vi "shift odd lines by.vi"(5 "calculate squared difference":bool, 7 "shift odd lines by":i32, 11 "frame in":dbl[][](array[numeric])) -> (2 "squared difference":dbl, 3 "shifted frame out":dbl[][](array[numeric]))   [LabVIEW 2012]
panel:
  out "corrected":T1(plugin-control)
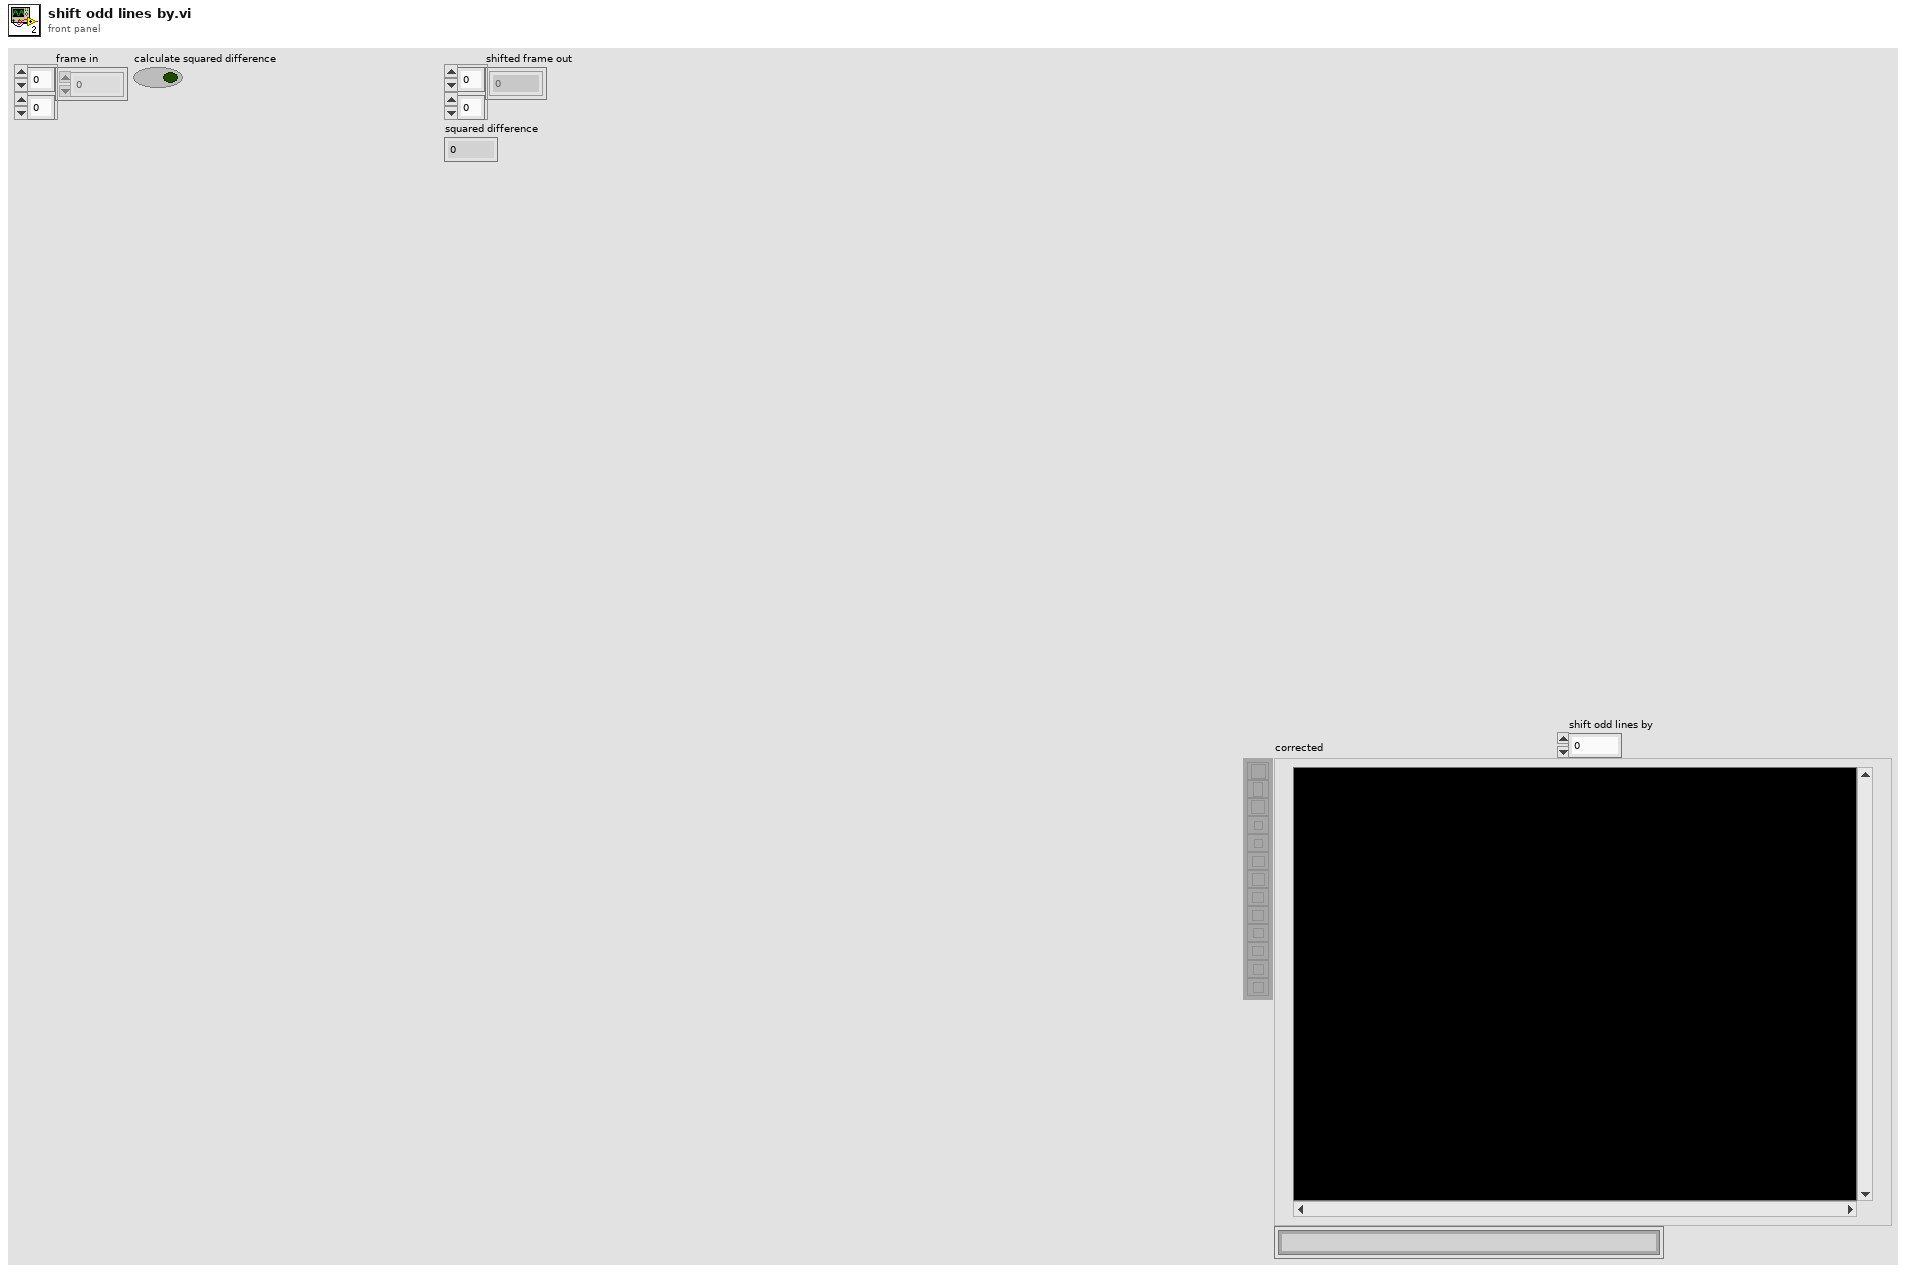
[diagram p1: front panel]
types:
  T1 = typedef "IMAQ Image.ctl" = refnum<image>
  T2 = typedef "Image Type" = u32
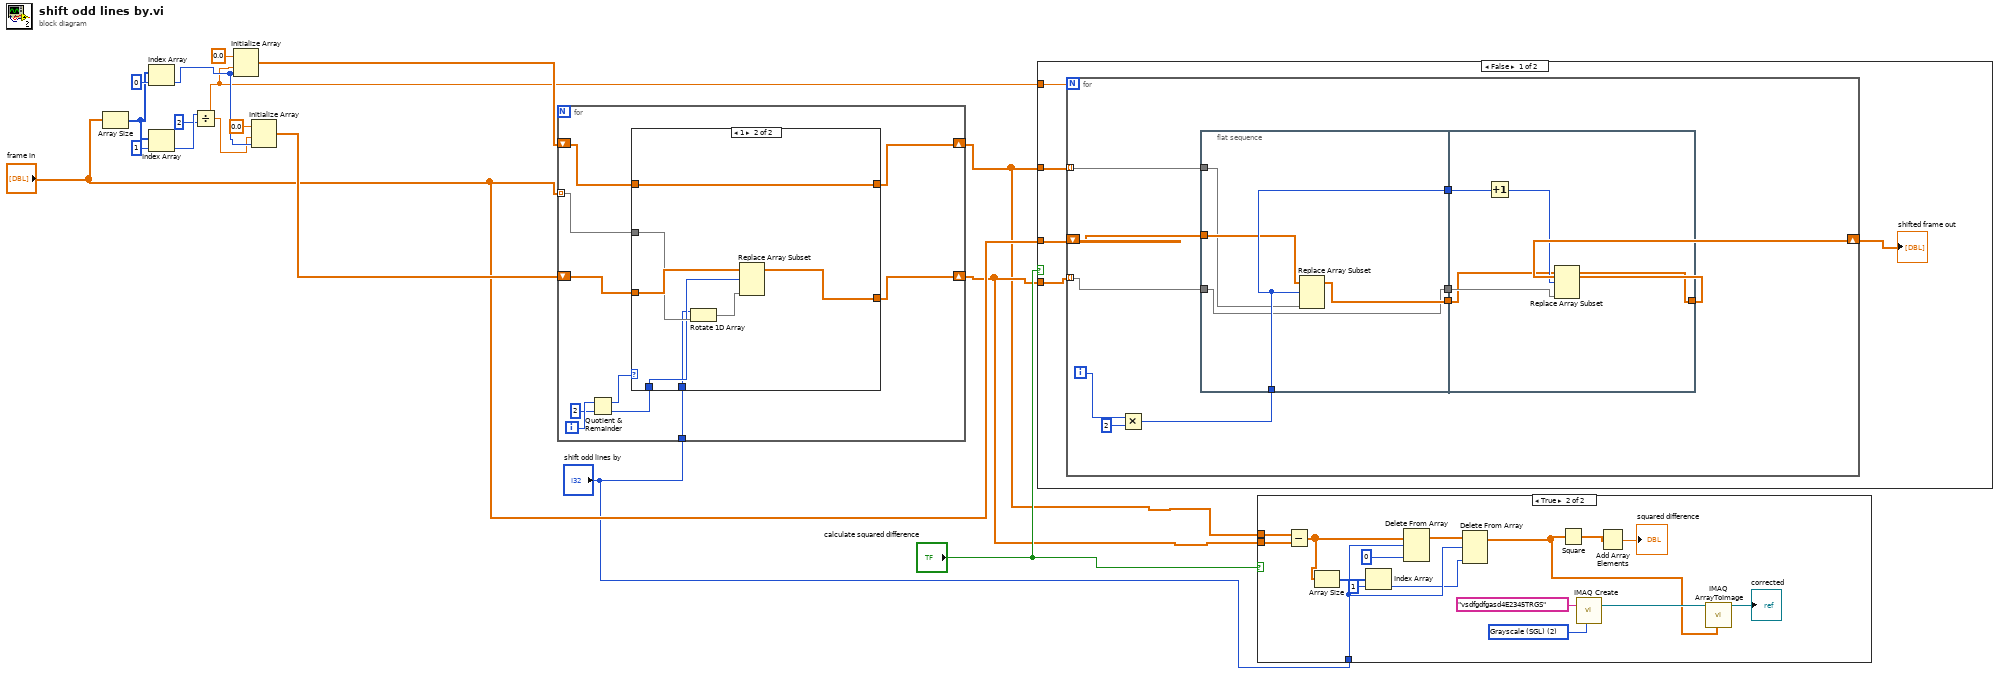
[diagram p0: block diagram]
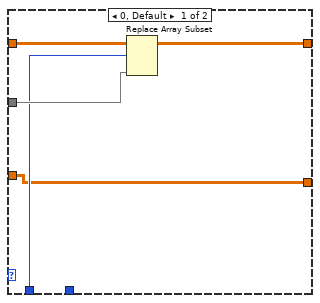
[diagram p4: hidden frame]
diagram:
  n1 = Array Size(array="frame in") -> (size(s)=w14:i32[])
  n2 = Index Array(array=w14, index=0) -> (element=w6:i32)
  n3 = Index Array(array=w14, index=1) -> (element=w13:i32)
  n4 = Divide(x=w13, y=2) -> (x/y=w5:dbl)
  n5 = Initialize Array(0.0 ("element"), w5, w6) -> (w11:dbl[][])
  n6 = Initialize Array(0.0 ("element"), w5, w6) -> (w8:dbl[][])
  n7 = for {
    tunnel: "frame in" -> [w23] mode=indexing
    shift-right: [w21] -> w1
    shift-left: w11 -> [w22]
    shift-right: [w18] -> w2
    shift-left: w8 -> [w19]
    tunnel: "shift odd lines by" -> [w17]
    i -> [w26]
    n8 = Quotient & Remainder(x=w26, y=2) -> (x-y*floor(x/y)=w24:i32, floor(x/y)=w20:i32)
    n9 = case shown="1" w24 {
      tunnel: w23 -> [w29 w37]
      tunnel: w22 -> [w31 w33]
      tunnel: [w30 w33] -> w21
      tunnel: w20 -> [w28 w35]
      tunnel: w19 -> [w27 w38]
      tunnel: [w27 w34] -> w18
      tunnel: w17 -> [_ w32]
      frame 0, Default {
        n10 = Replace Array Subset(array=w31, new element=w29, index (row)=w28) -> (w30:dbl[][])  [unwired: 1 in]
      }
      frame 1 {
        n11 = Rotate 1D Array(1:w37, 2:w32) -> (0:w36:dbl[])
        n12 = Replace Array Subset(array=w38, new element=w36, index (row)=w35) -> (w34:dbl[][])  [unwired: 1 in]
      }
    }
  }
  n13 = case shown="False" "calculate squared difference" {
    tunnel: "frame in" -> [w43 _]
    tunnel: w1 -> [w41 _]
    tunnel: w2 -> [w40 _]
    tunnel: w5 -> [w39 _]
    frame False {
      n14 = for {
        N: w39 -> [_]
        shift-right: [w49] -> w42
        shift-left: w43 -> [w53]
        tunnel: w41 -> [w50] mode=indexing
        tunnel: w40 -> [w52] mode=indexing
        i -> [w51]
        n15 = Multiply(x=w51, y=2) -> (x*y=w48:i32)
        n16 = flat-sequence {
          tunnel: w53 -> [w57]
          tunnel: [w55] -> w46
          tunnel: w52 -> [w54]
          tunnel: [w54] -> w45
          tunnel: w48 -> [w58]
          tunnel: [w58] -> w44
          tunnel: w50 -> [w56]
          tunnel: [w60] -> w49
          tunnel: w46 -> [w59]
          tunnel: w45 -> [w63]
          tunnel: w44 -> [w62]
          frame #0 {
            n17 = Replace Array Subset(array=w57, new element=w56, index (row)=w58) -> (w55:dbl[][])  [unwired: 1 in]
          }
          frame #1 {
            n18 = Increment(x=w62) -> (x+1=w61:i32)
            n19 = Replace Array Subset(array=w59, new element=w63, index (row)=w61) -> (w60:dbl[][])  [unwired: 1 in]
          }
        }
      }
      "shifted frame out" <- w42
    }
    frame True {
    }
  }
  n20 = case shown="True" "calculate squared difference" {
    tunnel: w1 -> [_ w78]
    tunnel: w2 -> [_ w77]
    tunnel: "shift odd lines by" -> [_ w69]
    frame False {
    }
    frame True {
      w75 = T2 2 items=["Grayscale (U8)", "Grayscale (I16)", "Grayscale (SGL)", "Complex (CSG)", "RGB (U32)", "HSL (U32)", "RGB (U64)", "Grayscale (U16)"] ("Image Type")
      n21 = Subtract(x=w78, y=w77) -> (x-y=w68:dbl[][])
      n22 = Array Size(array=w68) -> (size(s)=w66:i32[])
      n23 = Index Array(array=w66, index=1) -> (element=w64:i32)
      n24 = Delete From Array(array=w68, length=w69, index (col)=0 ("index (row)")) -> (array with subset deleted=w72:dbl[][])  [unwired: 1 in, 1 out]
      n25 = Delete From Array(array=w72, length=w69, index (col)=w64) -> (array with subset deleted=w70:dbl[][])  [unwired: 1 in, 1 out]
      n26 = Square(x=w70) -> (x^2=w79:dbl[][])
      n27 = call "IMAQ Create"("Image Name"="vsdfgdfgasd4E2345TRGS", "Image Type"=w75) -> ("New Image"=w73:T1)  [unwired: 3 in, 1 out]
      n28 = Add Array Elements(numeric array=w79) -> (sum=→"squared difference":dbl)
      n29 = call "IMAQ ArrayToImage"("Image Pixels (Float)"=w70, "Image"=w73) -> ("Image Out"=→"corrected":T1)  [unwired: 8 in, 1 out]
    }
  }
